vi "Read Group Name.vi"(8 "error in (no error)":errorcluster, 11 "Write Group Name Msg in":refnum<class "Write Group Name Msg.lvclass">) -> (0 "error out":errorcluster, 2 "Group Name":string, 3 "Write Group Name Msg out":refnum<class "Write Group Name Msg.lvclass">)   [LabVIEW 2015, in "Write Group Name Msg.lvclass"]
uses:
  Write Group Name Msg.lvclass
  Write Group Name Msg.lvclass/Write Group Name Msg.ctl
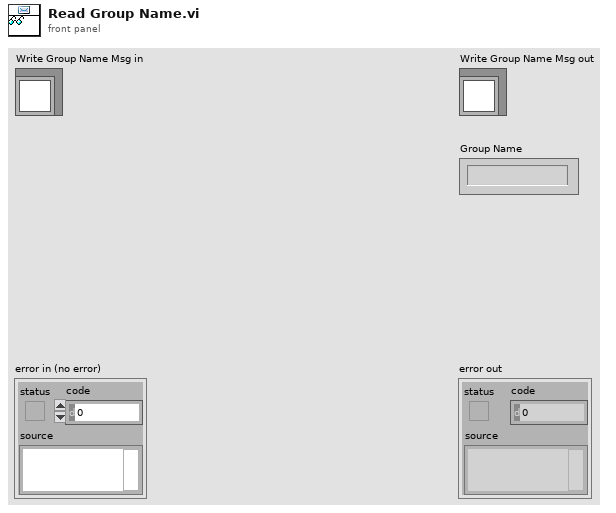
[diagram p1: front panel]
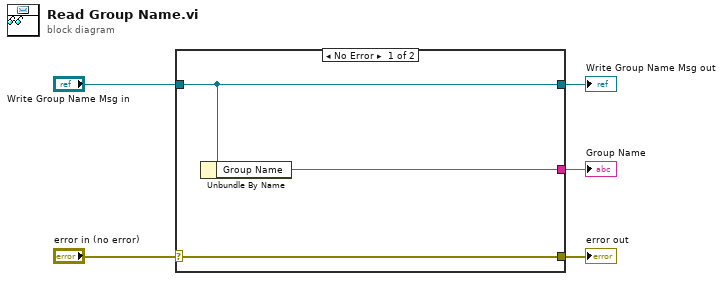
[diagram p0: block diagram]
diagram:
  n1 = case shown="No Error" "error in (no error)" {
    selector: "error in (no error)" -> [w8 w9]
    tunnel: [w8 w9] -> w4
    tunnel: [w7 w10] -> w2
    tunnel: "Write Group Name Msg in" -> [w7 w10]
    tunnel: [w6 _] -> w1
    frame No Error {
      n2 = Unbundle By Name(w7) -> ("Group Name"=w6:string)
    }
    frame Error {
    }
  }
  "error out" <- w4
  "Write Group Name Msg out" <- w2
  "Group Name" <- w1
